vi "niDTS WLAN INSTR RX Set niRfsgWlan Handle.vi"(8 "error in (no error)":errorcluster, 10 "InstDriver Handle in":T1, 11 "niDTS WLAN INSTR RX in":refnum<class "niDTS WLAN INSTR RX.lvclass">) -> (0 "error out":errorcluster, 3 "niDTS WLAN INSTR RX out":refnum<class "niDTS WLAN INSTR RX.lvclass">)   [LabVIEW 2015, in "niDTS WLAN.lvlib" / "niDTS WLAN INSTR RX.lvclass"]
uses:
  niDTS WLAN INSTR RX.lvclass
  RiviInstDriver/niRfsgWlan/Includes/niRfsgWlan INC Handle.ctl
  RiviInstDriver/niRfsgWlan/Objects/niRfsgWlan.lvclass
  niDTS WLAN INSTR RX.lvclass/niDTS WLAN INSTR RX.ctl
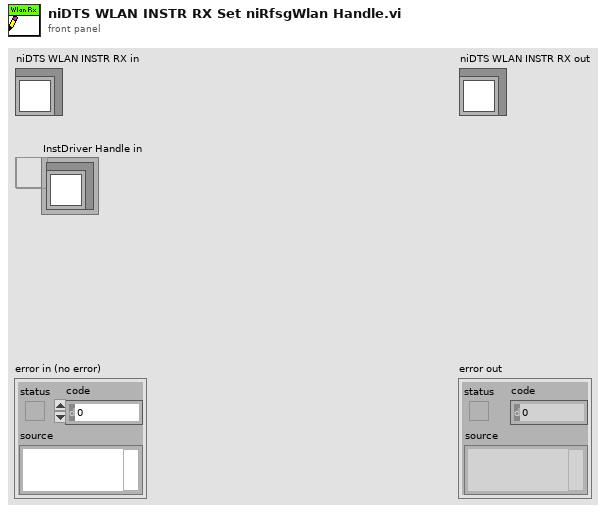
[diagram p1: front panel]
types:
  T1 = typedef "niRfsgWlan.lvclass/niRfsgWlan INC Handle.ctl" = refnum<data-value>
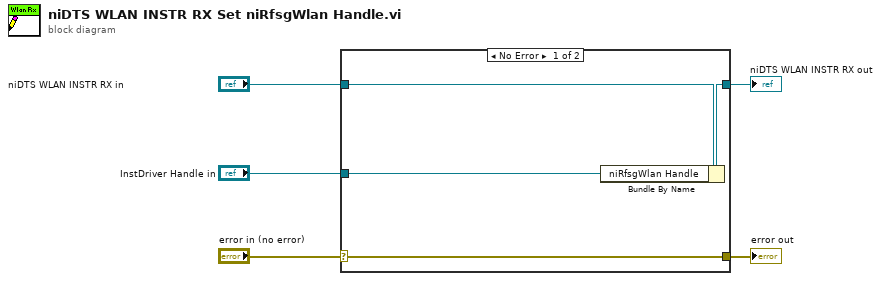
[diagram p0: block diagram]
diagram:
  n1 = case shown="No Error" "error in (no error)" {
    selector: "error in (no error)" -> [w9 w10]
    tunnel: [w9 w10] -> w4
    tunnel: [w7 w11] -> w2
    tunnel: "niDTS WLAN INSTR RX in" -> [w8 w11]
    tunnel: "InstDriver Handle in" -> [w6 _]
    frame No Error {
      n2 = Bundle By Name(cluster=w8, "niRfsgWlan Handle"=w6) -> (w7:refnum<class "niDTS WLAN INSTR RX.lvclass">)
    }
    frame Error {
    }
  }
  "error out" <- w4
  "niDTS WLAN INSTR RX out" <- w2
